vi "Publish If True.vi"(8 "error in (no error)":errorcluster, 9 "Data to Publish":bool, 10 "Datum Name":string, 11 "IModel in":refnum<class "IModel.lvclass">) -> (0 "error out":errorcluster, 3 "IModel out":refnum<class "IModel.lvclass">)   [LabVIEW 2017, in "IModel.lvlib" / "IModel.lvclass"]
doc: "Publish a Boolean value only if it is TRUE. This publication allows multiple actors or multiple sections of code to publish a flag that stays TRUE on the mediated bus until another actor intentionally handles it. (A simple many-to-one option for global flag setting)"
uses:
  IModel.lvclass
  C:/Git/mva-framework/Source/Framework/IObserver/IObserver/IObserver.lvclass
  <vilib>/ActorFramework/Actor/Actor.lvclass/Actor.ctl
  <vilib>/ActorFramework/Message Enqueuer/Message Enqueuer.lvclass/Message Enqueuer.ctl
  IModel.lvclass/IModel.ctl
  IMediator/PublishRequest/PublishRequest.lvclass/PublishRequest.ctl
  AbstractMessages/PreAddressedMsg/PreAddressedMsg.lvclass/PreAddressedMsg.ctl
  IMediator/IMediator Messages/Publish Msg/Publish Msg.lvclass/Publish Msg.ctl
  IMediator/IMediator Messages/Publish Msg/Send Pre-Addressed Publish.vi
  IObserver/IObserver/Read Unique ID.vi
  IMediator/PublishRequest/Pack Publish Request.vi
  <vilib>/ActorFramework/Message Enqueuer/Enqueue.vi
  AbstractMessages/PreAddressedMsg/Read Return Address.vi
  <vilib>/ActorFramework/Actor/Read Self Enqueuer.vi
  <vilib>/ActorFramework/Message Enqueuer/Init from Existing Queue.vi
  IObserver/IObserver/IObserver.lvclass
  C:/Program Files (x86)/National Instruments/LabVIEW 2017/vi.lib/ActorFramework/Actor/Actor.lvclass
  IMediator/IMediator Messages/Publish Msg/Publish Msg.lvclass
  C:/Git/mva-framework/Source/Framework/AbstractMessages/PreAddressedMsg/PreAddressedMsg.lvclass
  C:/Program Files (x86)/National Instruments/LabVIEW 2017/vi.lib/ActorFramework/Message/Message.lvclass
  <vilib>/ActorFramework/Message Priority Queue/Priority Enqueue.vi
  IMediator/PublishRequest/PublishRequest.lvclass
  <vilib>/ActorFramework/Message Enqueuer/Message Enqueuer.lvclass
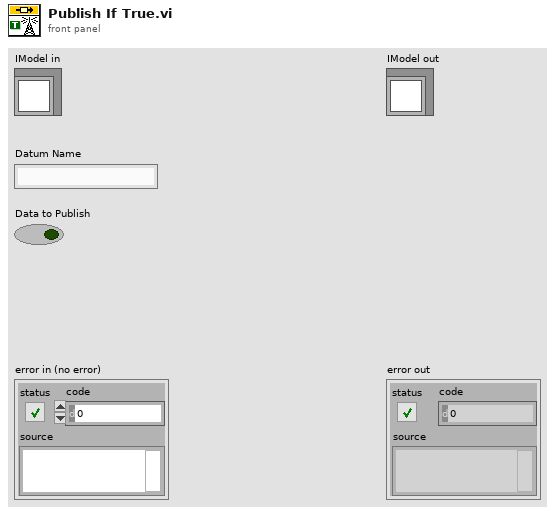
[diagram p1: front panel]
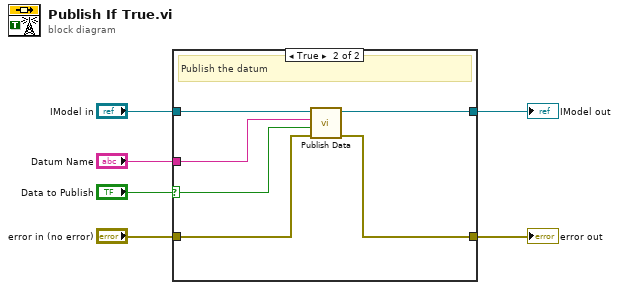
[diagram p0: block diagram]
diagram:
  n1 = case shown="True" "Data to Publish" {
    selector: "Data to Publish" -> [_ w9]
    tunnel: "IModel in" -> [w8 w14]
    tunnel: [w8 w13] -> w5
    tunnel: "error in (no error)" -> [w7 w12]
    tunnel: [w7 w11] -> w3
    tunnel: "Datum Name" -> [_ w10]
    frame False {
      # "...because it could clear prior state from the bus"
      # "Do not publish"
    }
    frame True {
      # "Publish the datum"
      n2 = call "Publish Data.vi"("error in (no error)"=w12, "Data to Publish"=w9, "Datum Name"=w10, "IModel in"=w14) -> ("error out"=w11:errorcluster, "IModel out"=w13:refnum<class "IModel.lvclass">)  [unwired: 6 in]
    }
  }
  "IModel out" <- w5
  "error out" <- w3
